vi "variantClusterByRef.vi"(8 "error in (no error)":errorcluster, 10 "MsgPack Variant":variant, 11 "Cluster Reference":refnum<vi>) -> (0 "error out":errorcluster, 3 "Cluster Reference (dup)":refnum<vi>)   [LabVIEW 2015, in "MsgPack.lvlib"]
uses:
  MsgPack.lvlib
  <vilib>/Utility/Data Type/NI_Data Type.lvlib
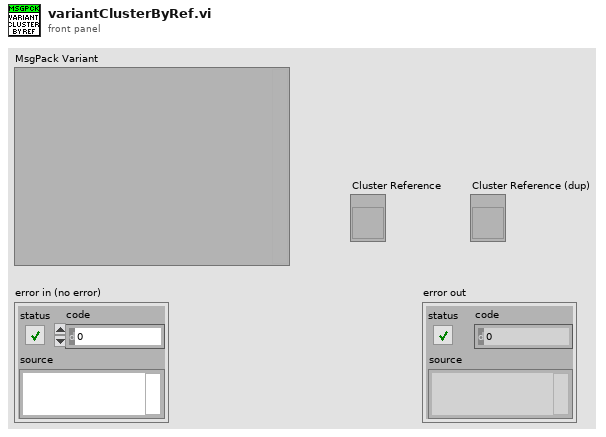
[diagram p1: front panel]
types:
  T1 = typedef "NI_Data Type.lvlib/Data Type.ctl" = enum8{"Invalid Type", "Void", "I8", "I16", "I32", "I64", "U8", "U16", "U32", "U64", "Single Float", "Double Float", "Extended Float", "Single Complex", "Double Complex", "Extended Complex", "Enum U8", "Enum U16", "Enum U32", "Enum U64", "Single Float With Unit", "Double Float With Unit", "Extended Float With Unit", "Single Complex with Unit", "Double Complex with Unit", "Extended Complex with Unit", "Boolean", "String", "Path", "Picture", "Tag", "Array", "Cluster", "Variant", "LV Variant", "Waveform", "Timestamp", "Digital Waveform", "Digital Data", "ExpressData", "Refnum", "External Data", "VI", "Poly VI", "LabVIEW Class Instance", "Fixed Point"}
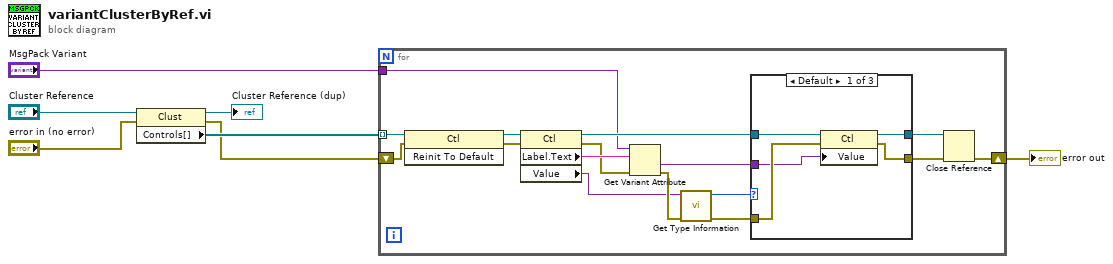
[diagram p0: block diagram]
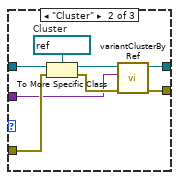
[diagram p2: hidden frame]
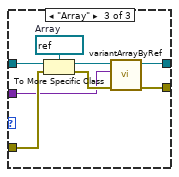
[diagram p3: hidden frame]
diagram:
  n1 = property class="Clust"(reference="Cluster Reference", error in="error in (no error)") -> (reference out=→"Cluster Reference (dup)":refnum<vi>, error out=w4:errorcluster, "Controls[]"=w5:refnum<vi>[])
  n2 = for {
    tunnel: w5 -> [w11] mode=indexing
    shift-right: [w12] -> w3
    shift-left: w4 -> [w9]
    tunnel: "MsgPack Variant" -> [w21]
    n3 = invoke class="Ctl" method="Reinit To Default"(reference=w11, error in=w9) -> (reference out=w10:refnum<vi>, error out=w8:errorcluster)  [unwired: 1 in, 1 out]
    n4 = property class="Ctl"(reference=w10, error in=w8) -> (reference out=w22:refnum<vi>, error out=w19:errorcluster, "Label.Text"=w20:string, "Value"=w17:variant)
    n5 = Get Variant Attribute(Variant=w21, name=w20, error in=w19) -> (value=w15:variant, error out=w18:errorcluster)  [unwired: 1 in, 2 out]
    n6 = call <vilib>:"Get Type Information.vi"("error in (no error)"=w18, "Variant"=w17) -> ("error out"=w16:errorcluster, "Type"=w23:T1)  [unwired: 5 in, 3 out]
    n7 = case shown="Default" w23 {
      tunnel: w22 -> [w28 w36 w44]
      tunnel: [w27 w32 w38] -> w13
      tunnel: w16 -> [w26 w35 w43]
      tunnel: w15 -> [w25 w30 w39]
      tunnel: [w24 w29 w37] -> w14
      frame Default {
        n8 = property class="Ctl"(reference=w28, error in=w26, "Value"=w25) -> (reference out=w24:refnum<vi>, error out=w27:errorcluster)
      }
      frame "Cluster" {
        w34 = refnum<vi> refnum  # Cluster
        n9 = To More Specific Class(target class=w34, reference=w36, error in=w35) -> (specific class reference=w31:refnum<vi>, error out=w33:errorcluster)
        n10 = call "variantClusterByRef.vi"("error in (no error)"=w33, "MsgPack Variant"=w30, "Cluster Reference"=w31) -> ("error out"=w32:errorcluster, "Cluster Reference (dup)"=w29:refnum<vi>)  [unwired: 7 in]
      }
      frame "Array" {
        w42 = refnum<vi> refnum  # Array
        n11 = To More Specific Class(target class=w42, reference=w44, error in=w43) -> (specific class reference=w41:refnum<vi>, error out=w40:errorcluster)
        n12 = call "variantArrayByRef.vi"("error in (no error)"=w40, "Variant"=w39, "Array Ref"=w41) -> ("error out"=w38:errorcluster, "Array Ref (dup)"=w37:refnum<vi>)  [unwired: 7 in]
      }
    }
    n13 = Close Reference(reference=w14, error in (no error)=w13) -> (error out=w12:errorcluster)
  }
  "error out" <- w3
